vi "FTW-Container-Value-Timestamp.vi"(0 "JSON":refnum<class "FTW-Container.lvclass">, 11 "error in":errorcluster) -> (4 "JSON out":refnum<class "FTW-Container.lvclass">, 8 "Value":timestamp format="%<%Y-%m-%d %H:%M:%S%03u>T", 15 "error out":errorcluster)   [LabVIEW 2015, in "FTW-Container.lvclass"]
uses:
  FTW-Container.lvclass
  FTW-Container.lvclass/FTW-Container.ctl
  <vilib>/Utility/Data Type/NI_Data Type.lvlib
panel:
  # "Inputs"
  # "Outputs"
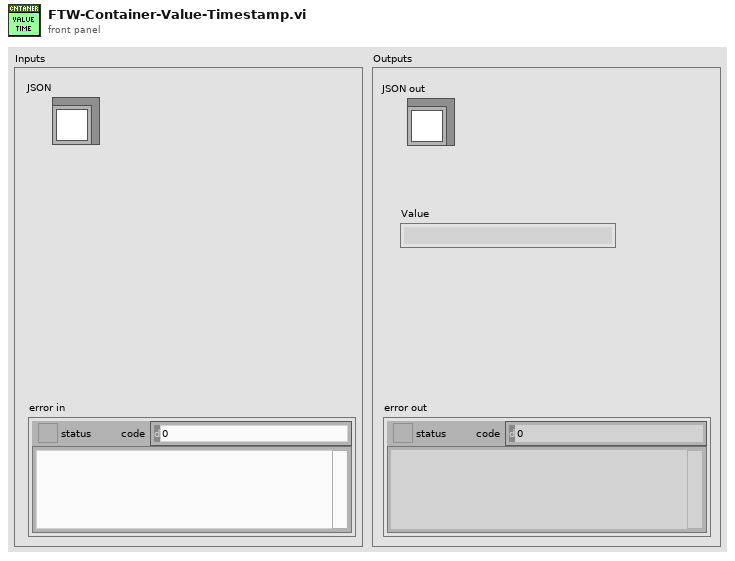
[diagram p1: front panel]
types:
  T1 = typedef "NI_Data Type.lvlib/Data Type.ctl" = enum8{"Invalid Type", "Void", "I8", "I16", "I32", "I64", "U8", "U16", "U32", "U64", "Single Float", "Double Float", "Extended Float", "Single Complex", "Double Complex", "Extended Complex", "Enum U8", "Enum U16", "Enum U32", "Enum U64", "Single Float With Unit", "Double Float With Unit", "Extended Float With Unit", "Single Complex with Unit", "Double Complex with Unit", "Extended Complex with Unit", "Boolean", "String", "Path", "Picture", "Tag", "Array", "Cluster", "Variant", "LV Variant", "Waveform", "Timestamp", "Digital Waveform", "Digital Data", "ExpressData", "Refnum", "External Data", "VI", "Poly VI", "LabVIEW Class Instance", "Fixed Point"}
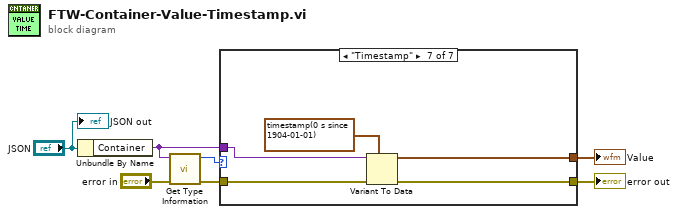
[diagram p0: block diagram]
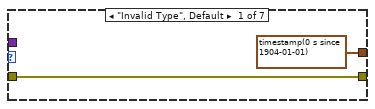
[diagram p2: hidden frame]
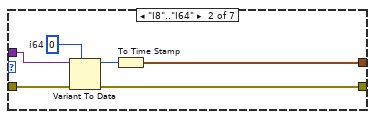
[diagram p3: hidden frame]
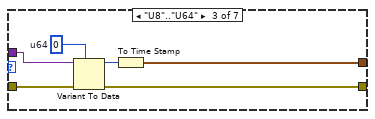
[diagram p4: hidden frame]
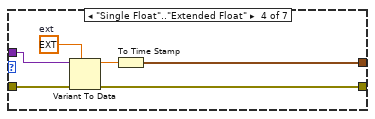
[diagram p5: hidden frame]
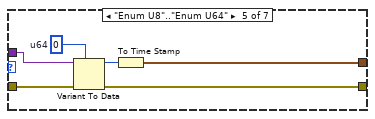
[diagram p6: hidden frame]
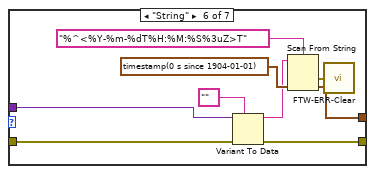
[diagram p7: hidden frame]
diagram:
  n1 = Unbundle By Name("JSON") -> ("Container"=w1:variant)
  n2 = call <vilib>:"Get Type Information.vi"("error in (no error)"="error in", "Variant"=w1) -> ("error out"=w4:errorcluster, "Type"=w3:T1)  [unwired: 5 in, 3 out]
  n3 = case shown="\"Timestamp\"" w3 {
    tunnel: w4 -> [w9 w14 w20 w26 w32 w38 w46]
    tunnel: w1 -> [_ w13 w19 w25 w31 w35 w45]
    tunnel: [w9 w12 w18 w24 w30 w37 w44] -> w6
    tunnel: [timestamp(0 s since 1904-01-01) w10 w16 w22 w28 w39 w43] -> w5
    frame "Invalid Type", Default {
    }
    frame "I8".."I64" {
      w15 = i64 0  # i64
      n4 = Variant To Data(error in=w14, type=w15, Variant=w13) -> (data=w11:i64, error out=w12:errorcluster)
      n5 = To Time Stamp(1:w11) -> (0:w10:timestamp)
    }
    frame "U8".."U64" {
      w21 = u64 0  # u64
      n6 = Variant To Data(error in=w20, type=w21, Variant=w19) -> (data=w17:u64, error out=w18:errorcluster)
      n7 = To Time Stamp(1:w17) -> (0:w16:timestamp)
    }
    frame "Single Float".."Extended Float" {
      w27 = ext 0.0  # ext
      n8 = Variant To Data(error in=w26, type=w27, Variant=w25) -> (data=w23:ext, error out=w24:errorcluster)
      n9 = To Time Stamp(1:w23) -> (0:w22:timestamp)
    }
    frame "Enum U8".."Enum U64" {
      w33 = u64 0  # u64
      n10 = Variant To Data(error in=w32, type=w33, Variant=w31) -> (data=w29:u64, error out=w30:errorcluster)
      n11 = To Time Stamp(1:w29) -> (0:w28:timestamp)
    }
    frame "String" {
      n12 = Variant To Data(error in=w38, type="" ("empty string"), Variant=w35) -> (data=w34:string, error out=w37:errorcluster)
      n13 = Scan From String(format string="%^<%Y-%m-%dT%H:%M:%S%3uZ>T", input string=w34, default 1=timestamp(0 s since 1904-01-01) ("LabVIEW Timestamp")) -> (error out=w42:errorcluster, output 1=w39:timestamp)  [unwired: 2 in, 2 out]
      n14 = call "FTW-ERR-Clear.vi"("error to snuff"=w42) -> ()  [unwired: 1 out]
    }
    frame "Timestamp" {
      n15 = Variant To Data(error in=w46, type=timestamp(0 s since 1904-01-01), Variant=w45) -> (data=w43:timestamp, error out=w44:errorcluster)
    }
  }
  "error out" <- w6
  "Value" <- w5
  "JSON out" <- "JSON"
